vi "Panel.vi"(11 "Cloned Panel in":refnum<class "Cloned Panel.lvclass">) -> ()   [LabVIEW 2020, in "Cloned UI.lvlib" / "Cloned Panel.lvclass"]
uses:
  Cloned Panel.lvclass
  C:/dev/LabVIEW/lv-oopanel/OOPanel/Panel/Panel.lvclass
  OOPanel/Panel/Panel.lvclass
panel:
  out "Iterations":i32
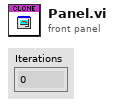
[diagram p1: front panel]
types:
  T1 = typedef "eventsource.ctl" = u32
  T2 = typedef "OOPanel.lvlib/Panel.lvclass/Visibility State.ctl" = enum16{"Idle", "Closed", "Hidden", "Visible", "Subpanel"}
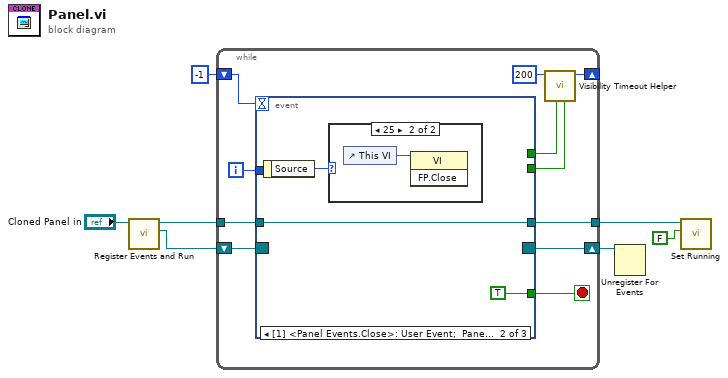
[diagram p0: block diagram]
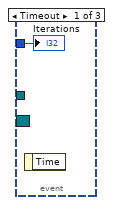
[diagram p2: hidden frame]
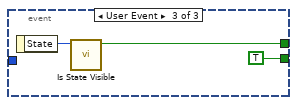
[diagram p4: hidden frame]
diagram:
  n1 = call "Register Events and Run.vi"("Panel in"="Cloned Panel in") -> ("Panel Event Reg"=w5:refnum<event-registration>, "Panel out"=w6:refnum<class "Cloned Panel.lvclass">)  [unwired: 8 in, 1 out]
  n2 = while {
    tunnel: w6 -> [w9]
    shift-right: [w17] -> w1
    shift-left: w5 -> [w18]
    shift-right: [w15] -> _
    shift-left: -1 -> [w14]
    tunnel: [w8] -> w3
    i -> [w11]
    stop <- w10 stop-if-true
    n3 = event shown="[1] <Panel Events.Close>: User Event;  Panel Close" {
      selector: w18 -> [_ _ _]
      dyn-events: [_ _ _] -> w17
      timeout: w14 -> [_ _ _]
      tunnel: [_ _ w25] -> w13
      tunnel: [_ _ TRUE] -> w12
      tunnel: w11 -> [w19 _ _]
      tunnel: [_ TRUE _] -> w10
      tunnel: w9 -> [_ w21 _]
      tunnel: [_ w21 _] -> w8
      event Timeout {
        n4 = event-data() -> ()  [unwired: 1 in, 1 out]
        "Iterations" <- w19
      }
      event User Event; Panel Close {
        n5 = event-data() -> ("Source"=w20:T1)  [unwired: 1 in]
        n6 = case shown="25" w20 {
          frame Default {
          }
          frame 25 {
            n7 = control-ref of="This VI"() -> (w23:refnum<vi>)
            n8 = invoke class="VI" method="FP.Close"(reference=w23) -> ()  [unwired: 2 in, 3 out]
          }
        }
      }
      event User Event {
        n9 = event-data() -> ("State"=w26:T2)  [unwired: 1 in]
        n10 = call "Is State Visible.vi"("Visibility"=w26) -> ("Visible"=w25:bool)  [unwired: 10 in]
      }
    }
    n11 = call "Visibility Timeout Helper.vi"("Update?"=w12, "Visible"=w13, "Visible Timeout mS"=200) -> ("Timeout"=w15:i32)  [unwired: 8 in]
  }
  n12 = Unregister For Events(event registration refnum=w1) -> ()  [unwired: 1 in, 1 out]
  n13 = call "Set Running.vi"("Running"=FALSE, "Panel in"=w3) -> ()  [unwired: 8 in, 2 out]
